vi "test_simple_threshold2.vi"() -> ()   [LabVIEW 2009]
doc: "Copyright (C) 2009, Stepan A. Baranov\nweb: http://www.OCTLab.org/\nemail: stepan@baranov.su"
uses:
  OCTLib.dll
panel:
  out "error out":errorcluster
  out "new_max":dbl
  out "new_min":dbl
  out "max":dbl
  out "min":dbl
  out "width":i32
  out "height":i32
  in  "Small/Big":bool
  out "loop #":i32
  out "RSM_STAT time":u32
  out "LabView time":u32
  out "RSM_STAT Array":dbl[][](array[numeric])
  out "LabView Array":dbl[][](array[numeric])
  in  "stop":bool
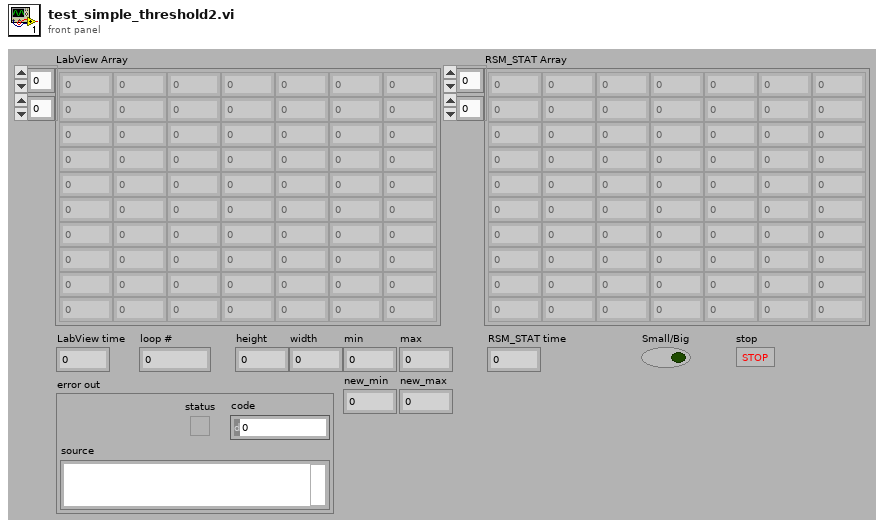
[diagram p1: front panel]
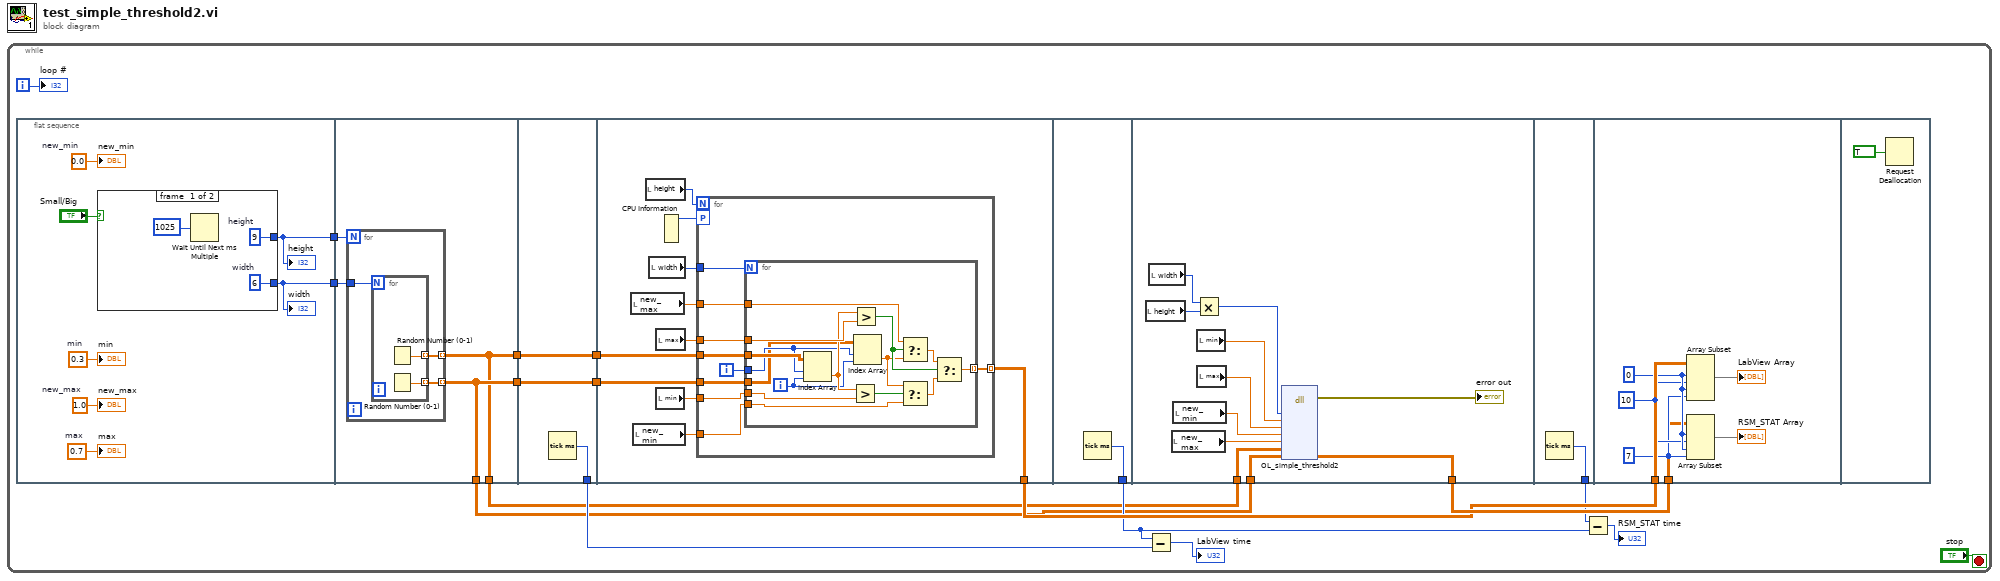
[diagram p0: block diagram]
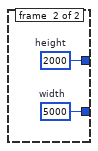
[diagram p2: hidden frame]
diagram:
  n1 = while {
    i -> [w9]
    stop <- "stop" stop-if-true
    n2 = flat-sequence {
      tunnel: [w23] -> w6
      tunnel: [w22] -> w5
      tunnel: [w31] -> w8
      tunnel: [w31] -> w7
      tunnel: w6 -> [w33]
      tunnel: w5 -> [w32]
      tunnel: [w30] -> w4
      tunnel: [w30] -> w2
      tunnel: [w41] -> w14
      tunnel: w7 -> [w39]
      tunnel: w4 -> [w40]
      tunnel: [w39] -> w3
      tunnel: [w40] -> w1
      tunnel: [w51] -> w15
      tunnel: w3 -> [w42]
      tunnel: w1 -> [w50]
      tunnel: [w76] -> w11
      tunnel: w8 -> [w87]
      tunnel: [w86] -> w16
      tunnel: w2 -> [w80]
      tunnel: [w88] -> w12
      tunnel: w16 -> [w89]
      tunnel: w15 -> [w95]
      frame #0 {
        w18 = 1.0  # new_max
        w19 = 0.0  # new_min
        w20 = 0.7  # max
        w21 = 0.3  # min
        n3 = case shown="True" "Small/Big" {
          tunnel: [w26 w29] -> w22
          tunnel: [w27 w28] -> w23
          frame #0 {
            w27 = 6  # width
            w26 = 9  # height
            n4 = Wait Until Next ms Multiple(millisecond multiple=u32 1025) -> ()  [unwired: 1 out]
          }
          frame #1 {
            w28 = 5000  # width
            w29 = 2000  # height
          }
        }
        "height" <- w22
        "width" <- w23
        "min" <- w21
        "max" <- w20
        "new_min" <- w19
        "new_max" <- w18
      }
      frame #1 {
        n5 = for {
          N: w32 -> [_]
          tunnel: w33 -> [w36]
          tunnel: [w35] -> w31 mode=indexing
          tunnel: [w34] -> w30 mode=indexing
          n6 = for {
            N: w36 -> [_]
            tunnel: [w38] -> w35 mode=indexing
            tunnel: [w37] -> w34 mode=indexing
            n7 = Random Number (0-1)() -> (number: 0 to 1=w37:dbl)
            n8 = Random Number (0-1)() -> (number: 0 to 1=w38:dbl)
          }
        }
      }
      frame #2 {
        n9 = Tick Count (ms)() -> (millisecond timer value=w41:u32)
      }
      frame #3 {
        n10 = local read "new_max"() -> (w44:dbl)
        n11 = local read "new_min"() -> (w43:dbl)
        n12 = local read "height"() -> (w49:i32)
        n13 = local read "width"() -> (w46:i32)
        n14 = local read "max"() -> (w48:dbl)
        n15 = local read "min"() -> (w47:dbl)
        n16 = CPU Information() -> (4:w45:i32)  [unwired: 3 out]
        n17 = for {
          N: w49 -> [_]
          tunnel: w48 -> [w57]
          tunnel: w47 -> [w56]
          tunnel: w46 -> [w55]
          tunnel: w50 -> [w60]
          tunnel: [w58] -> w51 mode=indexing
          workers-P: w45 -> [_]
          tunnel: w44 -> [w54]
          tunnel: w43 -> [w53]
          tunnel: w42 -> [w52]
          i -> [w59]
          n18 = for {
            N: w55 -> [_]
            tunnel: w59 -> [w63]
            tunnel: w57 -> [w74]
            tunnel: w56 -> [w73]
            tunnel: w60 -> [w75]
            tunnel: [w67] -> w58 mode=indexing
            tunnel: w54 -> [w66]
            tunnel: w53 -> [w65]
            tunnel: w52 -> [w62]
            i -> [w64]
            n19 = Index Array(array=w75, index (row)=w63, index (col)=w64) -> (element=w68:dbl)
            n20 = Greater?(x=w68, y=w73) -> (0:w72:bool)
            n21 = Greater?(x=w68, y=w74) -> (0:w71:bool)
            n22 = Index Array(array=w62, index (row)=w63, index (col)=w64) -> (element=w61:dbl)
            n23 = Select(t=w66, s=w71, f=w61) -> (s? t:f=w70:dbl)
            n24 = Select(t=w61, s=w72, f=w65) -> (s? t:f=w69:dbl)
            n25 = Select(t=w70, s=w71, f=w69) -> (s? t:f=w67:dbl)
          }
        }
      }
      frame #4 {
        n26 = Tick Count (ms)() -> (millisecond timer value=w76:u32)
      }
      frame #5 {
        n27 = local read "height"() -> (w82:i32)
        n28 = local read "width"() -> (w83:i32)
        n29 = local read "new_max"() -> (w79:dbl)
        n30 = local read "new_min"() -> (w78:dbl)
        n31 = Multiply(x=w83, y=w82) -> (x*y=w81:i32)
        n32 = local read "min"() -> (w85:dbl)
        n33 = local read "max"() -> (w84:dbl)
        n34 = dll-call lib="OCTLib.dll" fn="OL_simple_threshold2"("size"=w81, "min"=w85, "max"=w84, "new_min"=w78, "new_max"=w79, "ref"=w80, "data"=w87) -> (error out=→"error out":errorcluster, "data"=w86:dbl[][])  [unwired: 10 in, 1 out]
      }
      frame #6 {
        n35 = Tick Count (ms)() -> (millisecond timer value=w88:u32)
      }
      frame #7 {
        w92 = 10 ("length")
        w91 = 7 ("length")
        w93 = 0 ("index")
        n36 = Array Subset(array=w95, index (row)=w93, length (row)=w92, index (col)=w93, length (col)=w91) -> (→"LabView Array":dbl[][])
        n37 = Array Subset(array=w89, index (row)=w93, length (row)=w92, index (col)=w93, length (col)=w91) -> (→"RSM_STAT Array":dbl[][])
      }
      frame #8 {
        n38 = Request Deallocation(TRUE ("flag")) -> ()
      }
    }
    n39 = Subtract(x=w11, y=w14) -> (x-y=→"LabView time":u32)
    n40 = Subtract(x=w12, y=w11) -> (x-y=→"RSM_STAT time":u32)
    "loop #" <- w9
  }
